vi "Find Line Indent.vi"(0 "Functions in":T1[](array[typedef]), 1 "Indent Identifier":string="//", 11 "error in (no error)":errorcluster) -> (4 "Functions":T1[](array[typedef]), 15 "error out":errorcluster)   [LabVIEW 2019]
uses:
  Line Details.ctl
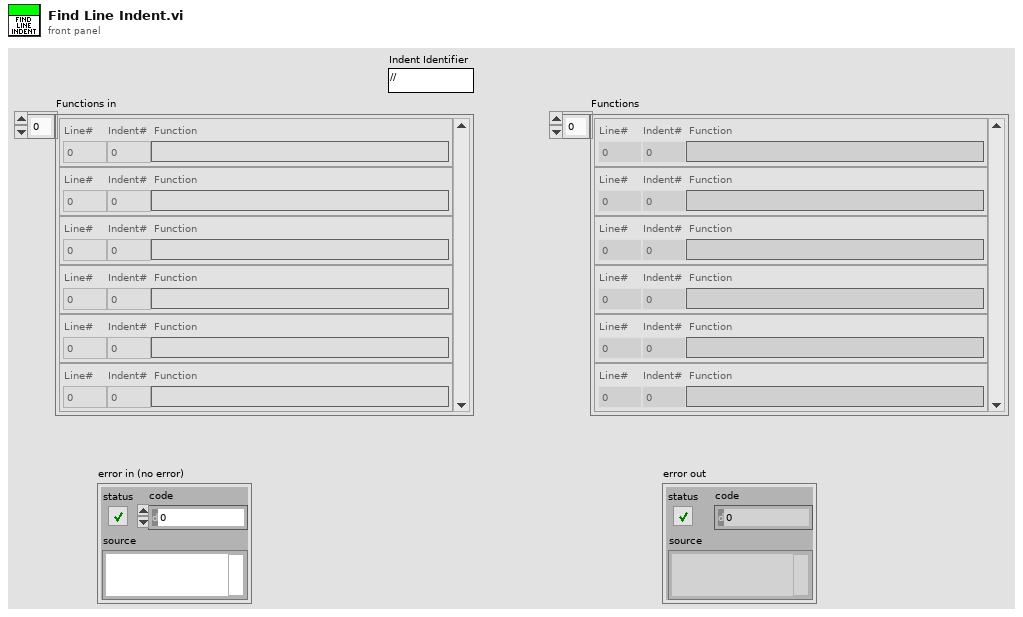
[diagram p1: front panel]
types:
  T1 = typedef "Line Details.ctl" = cluster{"Line#":i64, "Indent#":i64, "Function":string}
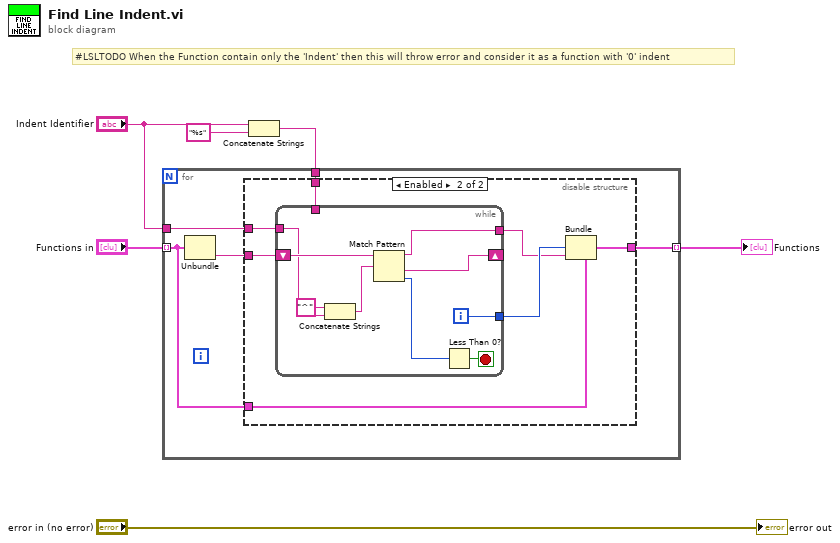
[diagram p0: block diagram]
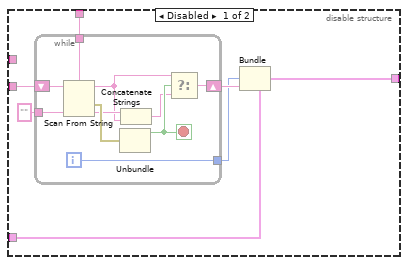
[diagram p2: hidden frame]
diagram:
  # "#LSLTODO When the Function contain only the 'Indent' then this will throw error and consider it as a function with '0' indent"
  n1 = Concatenate Strings("Indent Identifier", "%s" ("string")) -> (w4:string)
  n2 = for {
    tunnel: "Functions in" -> [w8] mode=indexing
    tunnel: w4 -> [w11]
    tunnel: [w10] -> w2 mode=indexing
    tunnel: "Indent Identifier" -> [w7]
    n3 = Unbundle(w8) -> ("Function"=w9:string)  [unwired: 2 out]
    n4 = disable-structure shown="Enabled" {
      disable-tunnel: w11 -> [w18 w34]
      disable-tunnel: [w17 w30] -> w10
      disable-tunnel: w9 -> [w15 w35]
      disable-tunnel: w8 -> [w14 w32]
      disable-tunnel: w7 -> [_ w33]
      frame Disabled {
        n5 = while {
          tunnel: w18 -> [w28]
          tunnel: [w26] -> w12
          tunnel: "" -> [w25]
          shift-right: [w21] -> w13
          shift-left: w15 -> [w24]
          i -> [w26]
          stop <- w23 stop-if-true
          n6 = Scan From String(format string=w28, input string=w24, default 1=w25) -> (remaining string=w19:string, error out=w27:errorcluster, output 1=w22:string)  [unwired: 2 in, 1 out]
          n7 = Unbundle(w27) -> ("status"=w23:bool)  [unwired: 2 out]
          n8 = Concatenate Strings(w22, w19) -> (w20:string)
          n9 = Select(t=w19, s=w23, f=w20) -> (s? t:f=w21:string)
        }
        n10 = Bundle(cluster=w14, "Indent#"=w12, "Function"=w13) -> (w17:T1)  [unwired: 1 in]
      }
      frame Enabled {
        n11 = while {
          shift-right: [w38] -> _
          shift-left: w35 -> [w44]
          tunnel: w34 -> [_]
          tunnel: w33 -> [w43]
          tunnel: [w36] -> w31
          tunnel: [w37] -> w29
          i -> [w36]
          stop <- w40 stop-if-true
          n12 = Concatenate Strings("^" ("string"), w43) -> (w42:string)
          n13 = Match Pattern(string=w44, regular expression=w42) -> (before substring=w37:string, after substring=w38:string, offset past match=w39:i32)  [unwired: 1 in, 1 out]
          n14 = Less Than 0?(x=w39) -> (x < 0?=w40:bool)
        }
        n15 = Bundle(cluster=w32, "Indent#"=w31, "Function"=w29) -> (w30:T1)  [unwired: 1 in]
      }
    }
  }
  "Functions" <- w2
  "error out" <- "error in (no error)"
